vi "test read.vi"() -> ()   [LabVIEW 2021]
panel:
  in  "error in (no error)":errorcluster
  in  "stop":bool
  out "error out":errorcluster
  out "data in":T1
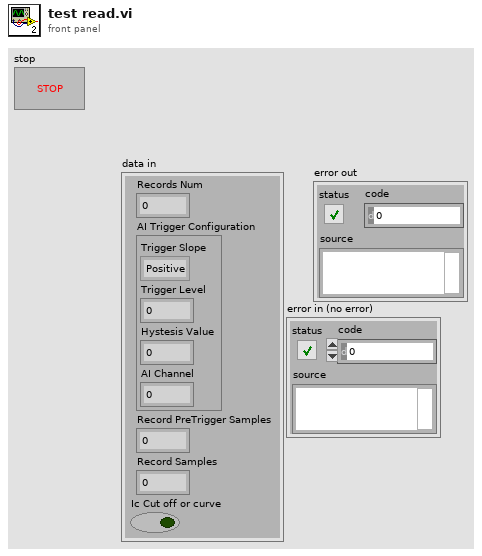
[diagram p1: front panel]
types:
  T1 = cluster{"Records Num":i32, "AI Trigger Configuration":cluster{"Trigger Slope":enum8{"Positive", "Negative"}, "Trigger Level":fxp<+/-,17,5>, "Hystesis Value":fxp<+,16,4>, "AI Channel":u8}, "Record PreTrigger Samples":u32, "Record Samples":u32, "Ic Cut off or curve":bool}
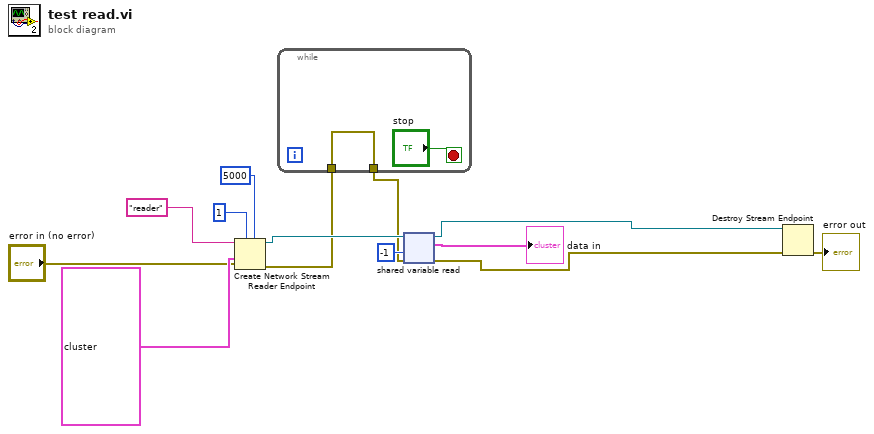
[diagram p0: block diagram]
diagram:
  n1 = Create Network Stream Reader Endpoint(5:5000 ("timeout in ms (-1)"), 7:1 ("reader buffer size"), 8:"error in (no error)", 9:T1 {"Records Num"=0, "AI Trigger Configuration"={"Trigger Slope"=enum."Positive", "Trigger Level"=0.0, "Hystesis Value"=0.0, "AI Channel"=0}, "Record PreTrigger Samples"=0, "Record Samples"=0, "Ic Cut off or curve"=FALSE} ("data in 2"), 11:"reader" ("reader name")) -> (0:w4:errorcluster, 3:w10:refnum<k21>)  [unwired: 2 in]
  n2 = while {
    tunnel: [w14] -> w3
    tunnel: w4 -> [w14]
    stop <- "stop" stop-if-true
  }
  n3 = shared-variable-read(w10, w3, -1 ("timeout ms (-1)")) -> (w7:refnum<k21>, w8:errorcluster, →"data in":T1)  [unwired: 1 out]
  n4 = Destroy Stream Endpoint(8:w8, 11:w7) -> (0:→"error out":errorcluster)
